vi "Service Request Enable Query.vi"(0 "VISA resource name":refnum<visa-resource-name>, 11 "error in (no error)":errorcluster) -> (4 "VISA resource name out":refnum<visa-resource-name>, 6 "Service Request Enable":T1, 15 "error out":errorcluster)   [LabVIEW 2016, in "APT 300XAC Series.lvlib"]
doc: "Queries the Service Request enable register. Returns the decimal value of binary-weighted sum of bits.\n\nThe Standard Event Register consists of the following 8 bits.\nBit 0: MSB = Measurement Summary Bit\nBit 1: not used\nBit 2: EAV = Error Available \nBit 3: QSB = Questionable Summary Bit\nBit 4: MAV = Message Available\nBit 5: ESB = Event Summary Bit \nBit 6: not used\nBit 7: OSB = Operation Summary Bit\n\nExample:\n\nIf the query returns the binary mask (00000101|bin=5|dec) then SRQ(Service Request) is generated using is MAV and EAV only."
uses:
  APT 300XAC Series.lvlib
panel:
  # "BIT 0 ,01H,(1)    MSB = Measurement Summary Bit\nBIT 1 ,02H,(2)    Not Used\nBIT 2, 04H,(4)    EAV = Error Available\nBIT 3, 08H,(8)    QSB = Questionable Summary Bit\nBIT 4, 10H,(16)  MAV = Message Available\nBIT 5, 20H,(32)  ESB = Event Summary Bit\nBIT 6, 40H,(64)  Not Used\nBIT 7, 80H,(128)OSB = Operation Summary Bit"
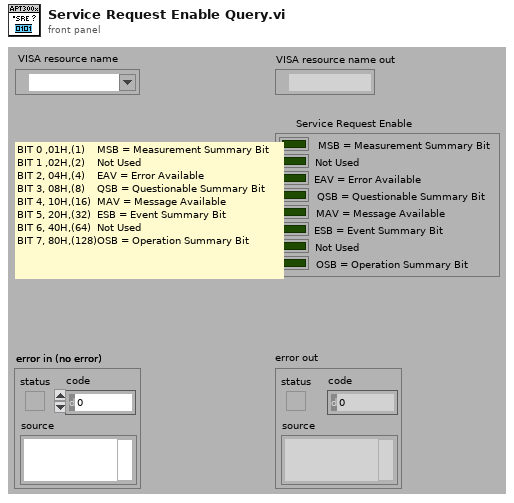
[diagram p1: front panel]
types:
  T1 = cluster{"MSB = Measurement Summary Bit":bool, "Not Used":bool, "EAV = Error Available":bool, "QSB = Questionable Summary Bit":bool, "MAV = Message Available":bool, "ESB = Event Summary Bit":bool, "Not Used":bool, "OSB = Operation Summary Bit":bool}
  T2 = cluster{"Boolean array[0]":bool, "Boolean array[1]":bool, "Boolean array[2]":bool, "Boolean array[3]":bool, "Boolean array[4]":bool, "Boolean array[5]":bool, "Boolean array[6]":bool, "Boolean array[7]":bool}
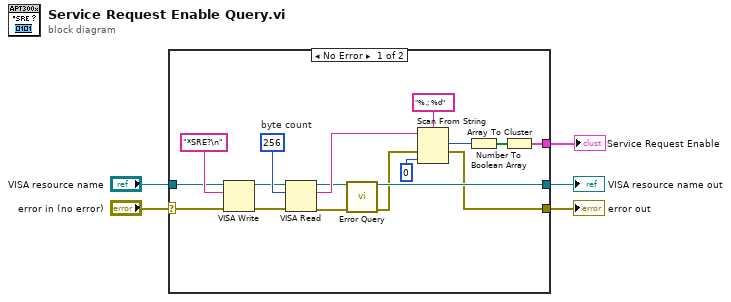
[diagram p0: block diagram]
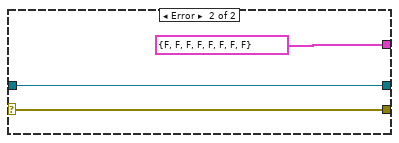
[diagram p2: hidden frame]
diagram:
  n1 = case shown="No Error" "error in (no error)" {
    selector: "error in (no error)" -> [w15 w25]
    tunnel: [w9 T2 {"Boolean array[0]"=FALSE, "Boolean array[1]"=FALSE, "Boolean array[2]"=FALSE, "Boolean array[3]"=FALSE, "Boolean array[4]"=FALSE, "Boolean array[5]"=FALSE, "Boolean array[6]"=FALSE, "Boolean array[7]"=FALSE} ("Boolean array")] -> w1
    tunnel: "VISA resource name" -> [w17 w24]
    tunnel: [w13 w24] -> w4
    tunnel: [w6 w25] -> w3
    frame No Error {
      w21 = u32 256  # byte count
      n2 = VISA Write(VISA resource name=w17, write buffer="*SRE?\n" ("Command to Send (empty)"), error in (no error)=w15) -> (VISA resource name out=w20:refnum<visa-resource-name>, error out=w19:errorcluster)  [unwired: 1 out]
      n3 = VISA Read(VISA resource name=w20, byte count=w21, error in (no error)=w19) -> (VISA resource name out=w12:refnum<visa-resource-name>, read buffer=w16:string, error out=w8:errorcluster)  [unwired: 1 out]
      n4 = call "Error Query.vi"("VISA resource name"=w12, "error in (no error)"=w8) -> ("VISA resource name out"=w13:refnum<visa-resource-name>, "error out"=w7:errorcluster)  [unwired: 10 in, 2 out]
      n5 = Scan From String(format string="%.; %d" ("Format String"), input string=w16, error in=w7, default 1=u8 0 ("default value 1")) -> (offset past scan=w10:u32, error out=w6:errorcluster)  [unwired: 2 in, 1 out]
      n6 = Number To Boolean Array(number=w10) -> (Boolean array=w11:bool[])
      n7 = Array To Cluster(array=w11) -> (cluster=w9:T2)
    }
    frame Error {
    }
  }
  "error out" <- w3
  "VISA resource name out" <- w4
  "Service Request Enable" <- w1
